vi "Test_WriteValue_ReadValue_ValueReturned.vi"(8 "error in (no error)":errorcluster, 11 "TestCase in":refnum<class "TestQueueTransport.lvclass">) -> (0 "error out":errorcluster, 3 "TestCase out":refnum<class "TestQueueTransport.lvclass">)   [LabVIEW 2017, in "TestQueueTransport.lvclass"]
uses:
  TestQueueTransport.lvclass
  Source/Concrete/QueueTransport/QueueTransport.lvclass/QueueTransport.ctl
  Source/Concrete/QueueTransport/QueueTransport.lvclass
  C:/Git/composed-transport/Source/ITransport/ITransport.lvclass
  <vilib>/Utility/error.llb/Error Cluster From Error Code.vi
  Source/ITransport/ITransport.lvclass
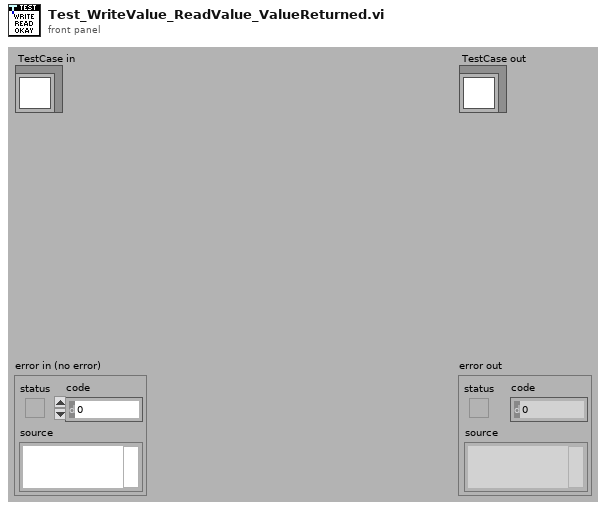
[diagram p1: front panel]
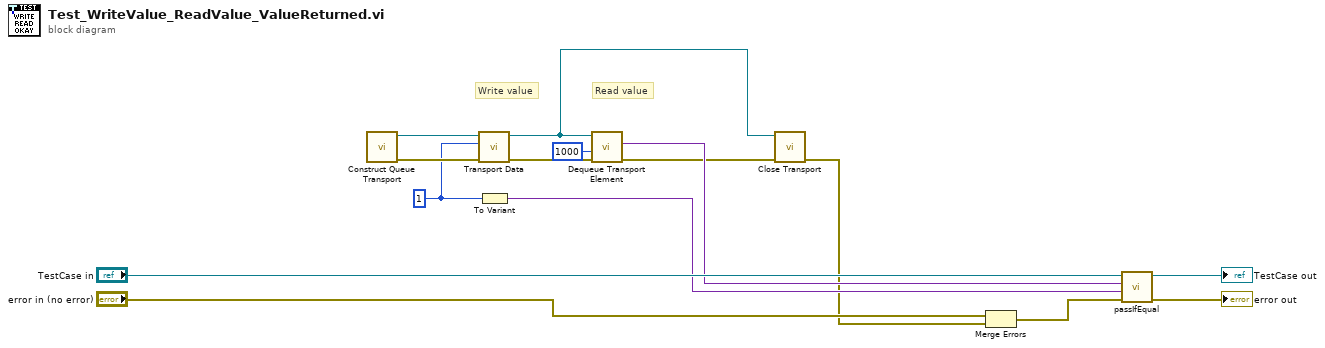
[diagram p0: block diagram]
diagram:
  w6 = 1
  # "Write value"
  # "Read value"
  n1 = call "Construct Queue Transport.vi"() -> ("error out"=w9:errorcluster, "QueueTransport"=w11:refnum<class "QueueTransport.lvclass">)  [unwired: 10 in]
  n2 = call "Transport Data.vi"("error in (no error)"=w9, "Value"=w6, "ITransport in"=w11) -> ("error out"=w8:errorcluster, "ITransport out"=w4:refnum<class "QueueTransport.lvclass">)  [unwired: 7 in]
  n3 = To Variant(anything=w6) -> (Variant=w5:variant)
  n4 = call "Dequeue Transport Element.vi"("error in (no error)"=w8, "Timeout In ms (-1)"=1000, "QueueTransport"=w4) -> ("error out"=w3:errorcluster, "Data"=w7:variant)  [unwired: 5 in, 2 out]
  n5 = call-dynamic "Close Transport.vi"("error in (no error)"=w3, "QueueTransport"=w4) -> ("error out"=w2:errorcluster)  [unwired: 9 in]
  n6 = Merge Errors("error in (no error)", w2) -> (w10:errorcluster)
  n7 = call-dynamic "passIfEqual.vi"("error in (no error)"=w10, "y"=w5, "x"=w7, "TestCase in"="TestCase in") -> ("error out"=→"error out":errorcluster, "TestCase out"=→"TestCase out":refnum<class "TestQueueTransport.lvclass">)  [unwired: 6 in]
